vi "Write Source filter.vi"(8 "Filter":string, 9 "Comparison type":T1, 10 "Field":T2, 11 "CDependencyInspection in":refnum<class "CDependencyInspection.lvclass">) -> (3 "CDependencyInspection out":refnum<class "CDependencyInspection.lvclass">)   [LabVIEW 2020, in "DependencyInspection.lvlib" / "CDependencyInspection.lvclass"]
uses:
  CDependencyInspection.lvclass
  CItemMatch/CItemMatch.lvclass
  CItemMatch/TypeDefs/Field.ctl
  CItemMatch/TypeDefs/ComparisonType.ctl
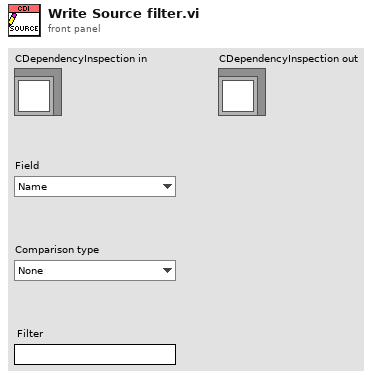
[diagram p1: front panel]
types:
  T1 = typedef "DependencyInspection.lvlib/CItemMatch.lvclass/ComparisonType.ctl" = enum16{"None", "Ends with", "Equals", "Not equal", "Starts with", "Contains", "Matches pattern"}
  T2 = typedef "DependencyInspection.lvlib/CItemMatch.lvclass/Field.ctl" = enum16{"Name", "Qualified name", "Path"}
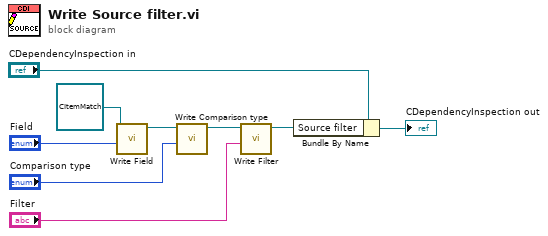
[diagram p0: block diagram]
diagram:
  n1 = call-dynamic "Write Field.vi"("Field"="Field", "CItemMatch in"=refnum<class "CItemMatch.lvclass"> refnum) -> ("CItemMatch out"=w4:refnum<class "CItemMatch.lvclass">)  [unwired: 9 in]
  n2 = call-dynamic "Write Comparison type.vi"("Comparison type"="Comparison type", "CItemMatch in"=w4) -> ("CItemMatch out"=w3:refnum<class "CItemMatch.lvclass">)  [unwired: 9 in]
  n3 = call-dynamic "Write Filter.vi"("Filter"="Filter", "CItemMatch in"=w3) -> ("CItemMatch out"=w2:refnum<class "CItemMatch.lvclass">)  [unwired: 9 in]
  n4 = Bundle By Name(cluster="CDependencyInspection in", "Source filter"=w2) -> (→"CDependencyInspection out":refnum<class "CDependencyInspection.lvclass">)
